vi "Get Unix Time.vi"() -> (0 "Unix Time":dbl format="%#.13f", 3 "Time Stamp (local)":timestamp)   [LabVIEW 2023]
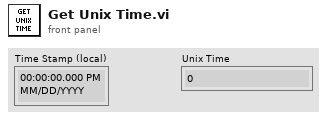
[diagram p1: front panel]
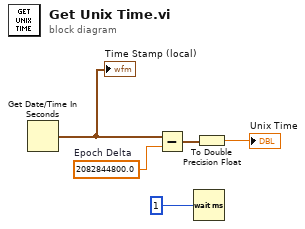
[diagram p0: block diagram]
diagram:
  w4 = 2082844800.0  # Epoch Delta
  n1 = Get Date/Time In Seconds() -> (seconds since 1Jan1904=w5:timestamp)
  "Time Stamp (local)" <- w5
  n2 = Subtract(x=w5, y=w4) -> (x-y=w3:timestamp)
  n3 = Wait (ms)(milliseconds to wait=u32 1) -> ()  [unwired: 1 out]
  n4 = To Double Precision Float(number=w3) -> (double precision float=→"Unix Time":dbl)
